vi "Read Device Identification.vi"(8 "error in":errorcluster, 9 "read device ID code":T2, 10 "object ID":u8, 11 "Modbus slave in":refnum<class "Modbus Slave.lvclass">) -> (0 "error out":errorcluster, 2 "objects":T1[](array[typedef]) {"Object ID" format="%x"}, 3 "Modbus slave out":refnum<class "Modbus Slave.lvclass">)   [LabVIEW 2012, in "Modbus Slave.lvclass"]
doc: "Reads Modbus object information stored on the device. This can include basic information, like manufacturer, additional standard items, or model-specific extended items. This function may take a large amount of time to execute, as it requires the transfer of a large quantity of binary data. Even on TCP/IP, this function is limited by the maximum defined size of a Modbus protocol data unit."
uses:
  Modbus Slave.lvclass
  Master Function Definition/Read Device ID code.ctl
  Data Model/Identification Parameters.ctl
  Modbus Slave.lvclass/Modbus Slave.ctl
  Data Model/Device Data Model.lvclass
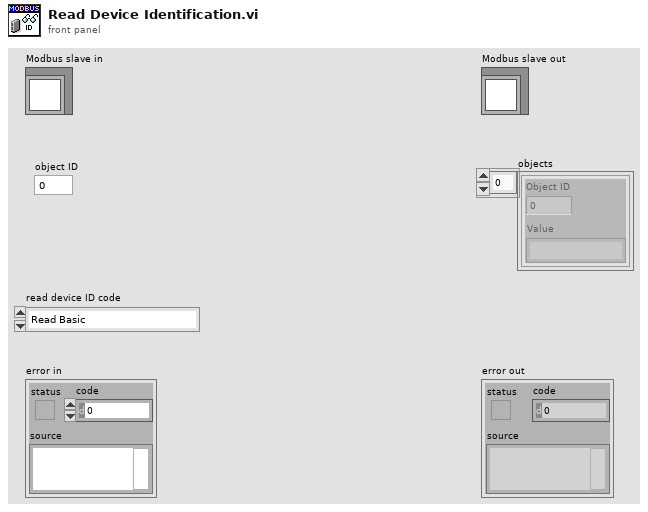
[diagram p1: front panel]
types:
  T1 = typedef "Device Data Model.lvclass/Identification Parameters.ctl" = cluster{"Object ID":u8, "Value":string}
  T2 = typedef "Device Data Model.lvclass/Read Device ID code.ctl" = enum8{"Read Basic", "Read Regular", "Read Extended", "Read Specific"}
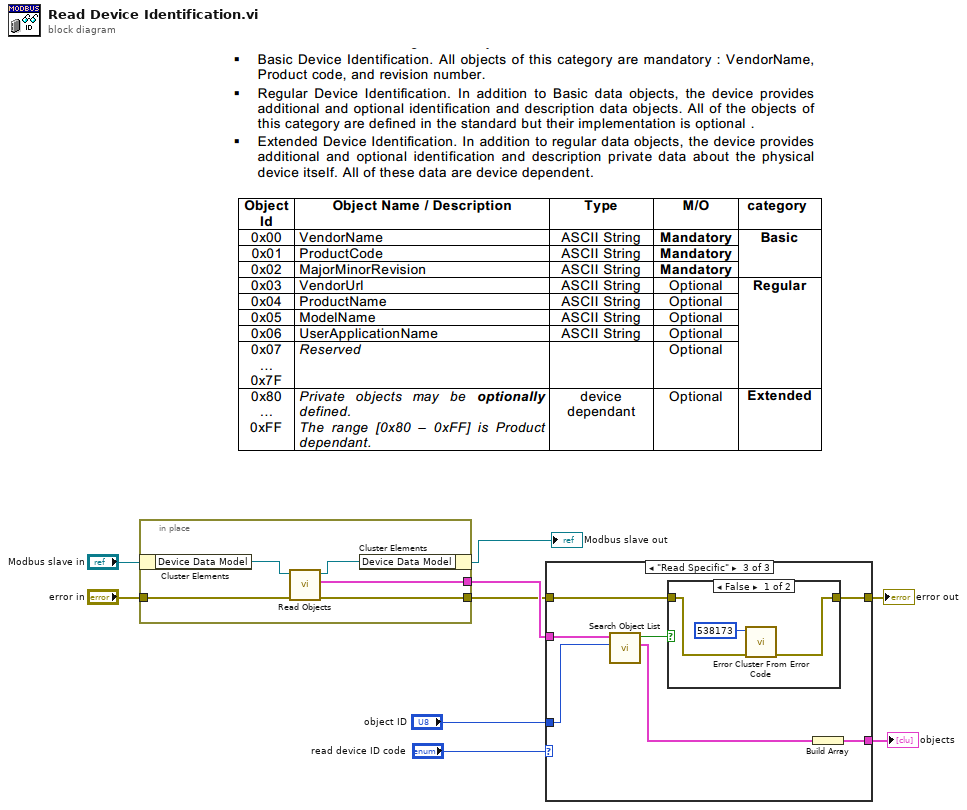
[diagram p0: block diagram]
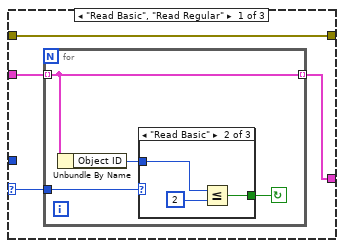
[diagram p2: hidden frame]
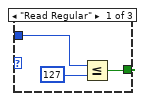
[diagram p3: hidden frame]
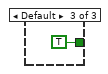
[diagram p4: hidden frame]
diagram:
  n1 = in-place {
    in-place-border: [w14] -> w7
    in-place-border: [w13] -> w1
    in-place-border: "error in" -> [w12]
    n2 = in-place-cluster #1("Modbus slave in") -> ("Device Data Model"=w11:refnum<class "Device Data Model.lvclass">)
    n3 = call-dynamic "Read Objects.vi"("error in"=w12, "device data model in"=w11) -> ("error out"=w13:errorcluster, "Objects"=w14:T1[], "device data model out"=w10:refnum<class "Device Data Model.lvclass">)  [unwired: 7 in]
    n4 = in-place-cluster #1("Device Data Model"=w10) -> (→"Modbus slave out":refnum<class "Modbus Slave.lvclass">)
  }
  n5 = case shown="\"Read Specific\"" "read device ID code" {
    selector: "read device ID code" -> [w15 _ _]
    tunnel: w7 -> [w17 w30 w38]
    tunnel: w1 -> [w18 w31 w33]
    tunnel: "object ID" -> [_ _ w37]
    tunnel: [w16 w30 w34] -> w4
    tunnel: [w18 w31 w32] -> w3
    frame "Read Basic", "Read Regular" {
      n6 = for {
        tunnel: w17 -> [w20] mode=indexing
        tunnel: [w20] -> w16 mode=indexing
        tunnel: w15 -> [w22]
        stop <- w21 continue-if-true
        n7 = Unbundle By Name(w20) -> ("Object ID"=w19:u8)
        n8 = case shown="\"Read Basic\"" w22 {
          tunnel: w19 -> [w25 w28 _]
          tunnel: [w23 w26 TRUE] -> w21
          frame "Read Regular" {
            n9 = Less Or Equal?(x=w25, y=u8 127) -> (x <= y?=w23:bool)
          }
          frame "Read Basic" {
            n10 = Less Or Equal?(x=w28, y=u8 2) -> (x <= y?=w26:bool)
          }
          frame Default {
          }
        }
      }
    }
    frame "Read Extended" {
    }
    frame "Read Specific" {
      n11 = call "Search Object List.vi"("Object ID"=w37, "Objects"=w38) -> ("Object"=w35:T1, "Found?"=w36:bool)  [unwired: 7 in, 1 out]
      n12 = case shown="False" w36 {
        tunnel: w33 -> [w40 w42]
        tunnel: [w41 w42] -> w32
        frame False {
          n13 = call <vilib>:"Error Cluster From Error Code.vi"("error in (no error)"=w40, "error code (0)"=538173) -> ("error out"=w41:errorcluster)  [unwired: 7 in]
        }
        frame True {
        }
      }
      n14 = Build Array(w35) -> (w34:T1[])
    }
  }
  "error out" <- w3
  "objects" <- w4
